vi "SOLICITAR_DIRECCION.vi"(8 "error in (no error)":errorcluster, 10 "BASE_DE_DATOS":string, 11 "DATABASE in":refnum<class "DATABASE.lvclass">) -> (0 "error out":errorcluster, 3 "DATABASE out":refnum<class "DATABASE.lvclass">)   [LabVIEW 2019, in "DATABASE.lvlib" / "DATABASE.lvclass"]
uses:
  DATABASE.lvclass
  DATABASE.lvclass/DATABASE.ctl
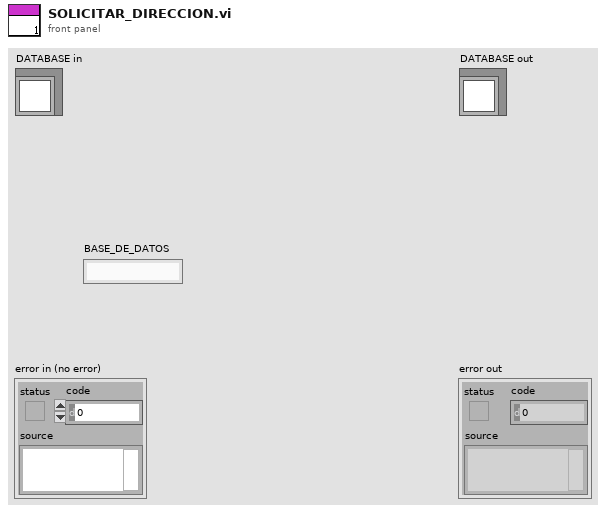
[diagram p1: front panel]
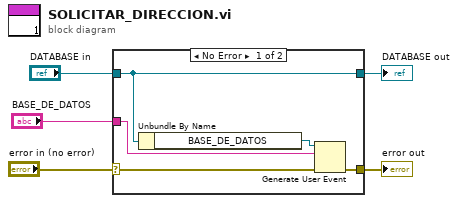
[diagram p0: block diagram]
diagram:
  n1 = case shown="No Error" "error in (no error)" {
    selector: "error in (no error)" -> [w7 w12]
    tunnel: [w6 w12] -> w4
    tunnel: [w10 w11] -> w2
    tunnel: "DATABASE in" -> [w10 w11]
    tunnel: "BASE_DE_DATOS" -> [w8 _]
    frame No Error {
      n2 = Unbundle By Name(w10) -> ("BASE_DE_DATOS"=w9:refnum<user-event>)
      n3 = Generate User Event(user event=w9, event data cluster=w8, error in=w7) -> (error out=w6:errorcluster)  [unwired: 1 in, 1 out]
    }
    frame Error {
    }
  }
  "error out" <- w4
  "DATABASE out" <- w2
